vi "Set Panes to Origins.vi"(8 "error in (no error)":errorcluster, 11 "IViewManager In":refnum<class "IViewManager.lvclass">) -> (0 "error out":errorcluster, 3 "IViewManager Out":refnum<class "IViewManager.lvclass">)   [LabVIEW 2015, in "IViewManager.lvlib" / "IViewManager.lvclass"]
uses:
  IViewManager.lvclass
  IViewManager.lvclass/IViewManager.ctl
  <vilib>/ActorFramework/Message Enqueuer/Message Enqueuer.lvclass/Message Enqueuer.ctl
  <vilib>/ActorFramework/Message Enqueuer/Enqueue.vi
  <vilib>/ActorFramework/Message Priority Queue/Priority Enqueue.vi
  IViewable/IViewable/IViewable.lvclass
  IViewable/IViewable Messages/Set Panes to Origins Msg/Set Panes to Origins Msg.lvclass
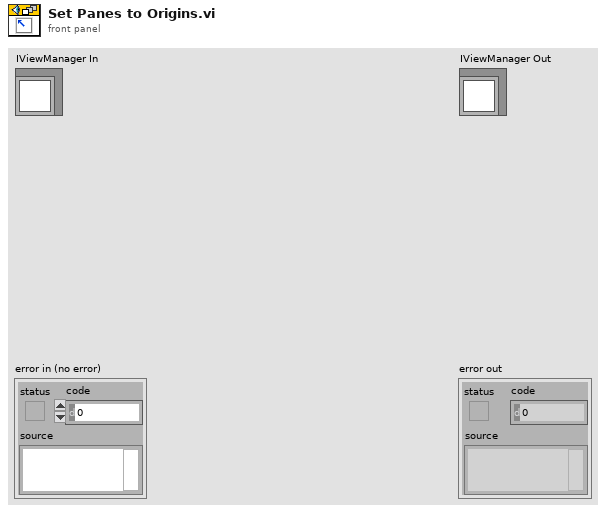
[diagram p1: front panel]
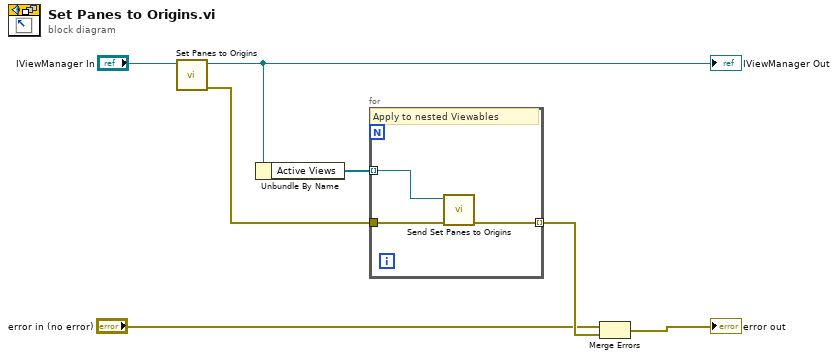
[diagram p0: block diagram]
diagram:
  n1 = call-parent "Set Panes to Origins.vi"("IViewable In"="IViewManager In") -> ("error out"=w7:errorcluster, "IViewable Out"=w5:refnum<class "IViewManager.lvclass">)  [unwired: 9 in]
  "IViewManager Out" <- w5
  n2 = Unbundle By Name(w5) -> ("Active Views"=w3:refnum<class "Message Enqueuer.lvclass">[])
  n3 = for {
    tunnel: w3 -> [w10] mode=indexing
    tunnel: w7 -> [w9]
    tunnel: [w8] -> w4 mode=indexing
    # "Apply to nested Viewables"
    n4 = call "Send Set Panes to Origins.vi"("error in (no error)"=w9, "Message Enqueuer"=w10) -> ("error out"=w8:errorcluster)  [unwired: 8 in, 1 out]
  }
  n5 = Merge Errors("error in (no error)", w4) -> (→"error out":errorcluster)
